vi "Start USB High-Speed Data Communication.vi"(0 "Device ID":i32, 1 "Max Buffer Size":u32, 9 "Start Req":T1={"High-Speed Comm Start Pos"=0, "Read Profile Cnt"=0, "High-Speed Receive Ratio"=16} {"High-Speed Receive Ratio" items=["LOWEST"=0, "LOW"=16, "MIDDLE"=17, "HIGH"=18, "HIGHEST"=32]; "High-Speed Comm Start Pos" items=["SEND COMPLETE POS", "OLDEST", "NEXT"]}, 11 "error in (no error)":errorcluster) -> (4 "Device ID out":i32, 6 "Return Code":i32, 15 "error out":errorcluster)   [LabVIEW 2014, in "Keyence LJ-V7000.lvlib"]
uses:
  Keyence LJ-V7000.lvlib
  Clusters/High-Speed Comm Start Req.ctl
  constant/High-Speed Comm Start Pos.ctl
  constant/High-Speed Receive Ratio.ctl
panel:
  # "(c) 2012 KEYENCE CORPORATION.  ALL RIGHTS RESERVED."
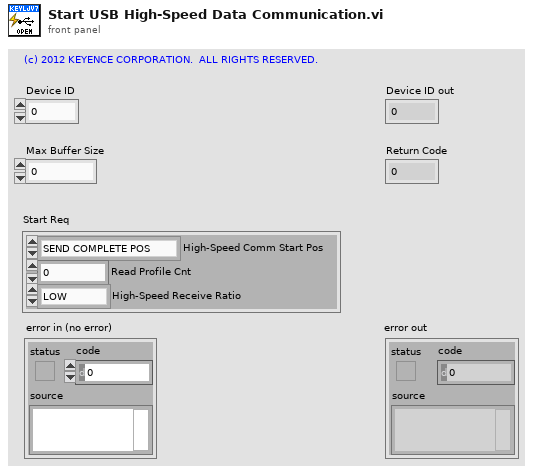
[diagram p1: front panel]
types:
  T1 = typedef "Keyence LJ-V7000.lvlib/High-Speed Comm Start Req.ctl" = cluster{"High-Speed Comm Start Pos":T2, "Read Profile Cnt":u32, "High-Speed Receive Ratio":T3}
  T2 = typedef "Keyence LJ-V7000.lvlib/High-Speed Comm Start Pos.ctl" = u8
  T3 = typedef "Keyence LJ-V7000.lvlib/High-Speed Receive Ratio.ctl" = u8
  T4 = cluster{"High-Speed Comm Start Pos":T2, "reserved":u8, "reserved":u8, "reserved":u8}
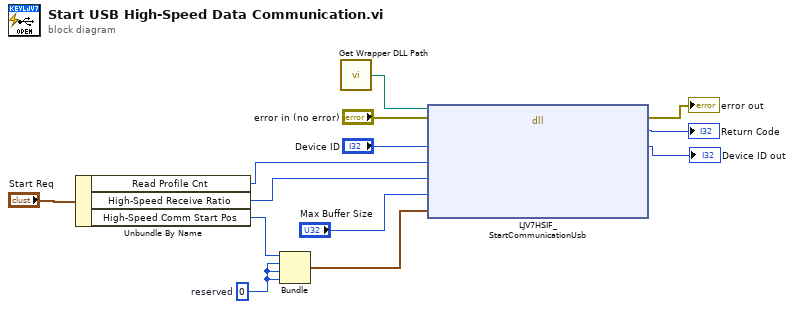
[diagram p0: block diagram]
diagram:
  w3 = u8 0  # reserved
  n1 = Unbundle By Name("Start Req") -> ("Read Profile Cnt"=w6:u32, "High-Speed Receive Ratio"=w5:T3, "High-Speed Comm Start Pos"=w4:T2)
  n2 = Bundle("High-Speed Comm Start Pos"=w4, "reserved"=w3, "reserved"=w3, "reserved"=w3) -> (w2:T4)  [unwired: 1 in]
  n3 = call "Get Wrapper DLL Path.vi"() -> ("Wrapper DLL Path"=w8:path)  [unwired: 1 in]
  n4 = dll-call lib="C:/Program Files/National Instruments/LabVIEW 2011/instr.lib/Keyence LJ-V7000/LJV7_HighSpeedWrapper.dll" fn="LJV7HSIF_StartCommunicationUsb"(path in=w8, error in="error in (no error)", "lDeviceId"="Device ID", "dwReqProfileCnt"=w6, "byReceiveRatio"=w5, "dwMaxBufferSize"="Max Buffer Size", "pReq"=w2) -> (error out=→"error out":errorcluster, "lRetCode"=→"Return Code":i32, "lDeviceId"=→"Device ID out":i32)  [unwired: 5 in, 1 out]
